vi "T7MOD_Write_UINT32_Registers.vi"(7 "UINT32 to Write":u32[](array[numeric]), 8 "error in":errorcluster, 9 "Starting Address":i32=55120, 10 "Remote Port":u16=502, 11 "Remote IP Address":string="192.168.1.15") -> (0 "error out":errorcluster, 1 "Written At":timestamp)   [LabVIEW 2018]
panel:
  # "Input"
  # "TCP Parameters"
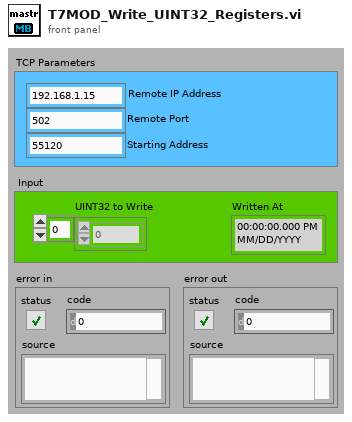
[diagram p1: front panel]
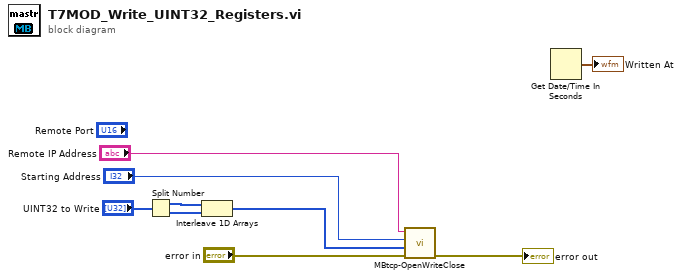
[diagram p0: block diagram]
diagram:
  n1 = Split Number(x="UINT32 to Write") -> (hi(x)=w7:u16[], lo(x)=w6:u16[])
  n2 = Interleave 1D Arrays(w7, w6) -> (w3:u16[])
  n3 = call "MBtcp-OpenWriteClose.vi"("error in (no error)"="error in", "Values"=w3, "RegisterAddr"="Starting Address", "IP Address(:port)"="Remote IP Address") -> ("error out"=→"error out":errorcluster)  [unwired: 7 in]
  n4 = Get Date/Time In Seconds() -> (seconds since 1Jan1904=→"Written At":timestamp)
